vi "visualization_sub_analog.vi"(10 "Latest?":bool, 11 "Instance":i32) -> (2 "ADC_Array":dbl[](array[numeric]), 3 "Analog Data Cluster":T1, 5 "dataToRead?":bool)   [LabVIEW 2022 SP3]
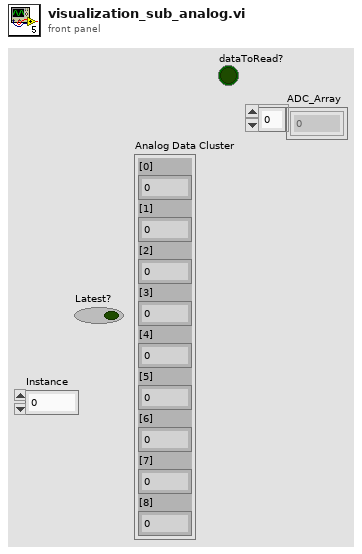
[diagram p1: front panel]
types:
  T1 = cluster{"[0]":dbl, "[1]":dbl, "[2]":dbl, "[3]":dbl, "[4]":dbl, "[5]":dbl, "[6]":dbl, "[7]":dbl, "[8]":dbl}
  T2 = cluster{"ADC_Array[0]":dbl, "ADC_Array[1]":dbl, "ADC_Array[2]":dbl, "ADC_Array[3]":dbl, "ADC_Array[4]":dbl, "ADC_Array[5]":dbl, "ADC_Array[6]":dbl, "ADC_Array[7]":dbl, "ADC_Array[8]":dbl}
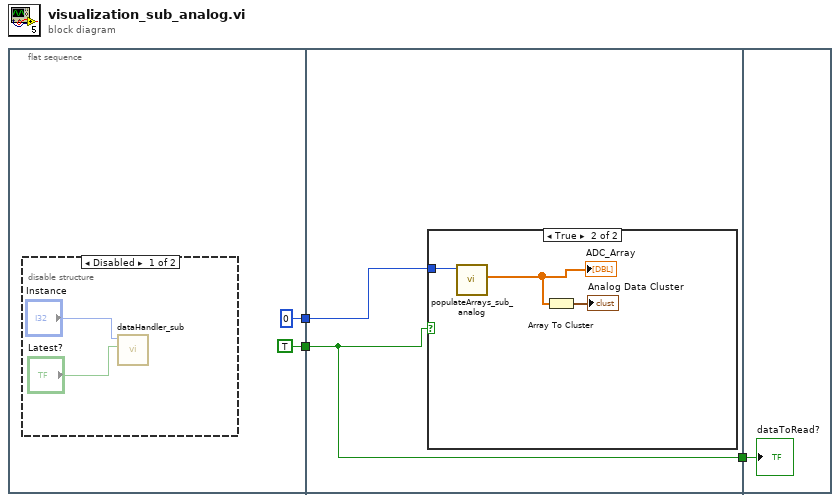
[diagram p0: block diagram]
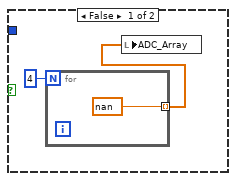
[diagram p3: hidden frame]
diagram:
  n1 = flat-sequence {
    tunnel: [0 ("Instance")] -> w3
    tunnel: [TRUE ("dataToRead?")] -> w2
    tunnel: w3 -> [w9]
    tunnel: w2 -> [w8]
    tunnel: [w8] -> w1
    tunnel: w1 -> [w16]
    frame #0 {
      n2 = disable-structure shown="Disabled" {
        frame Disabled {
          n3 = call "dataHandler_sub.vi"("Instance"="Instance", "Latest?"="Latest?") -> ()  [unwired: 7 in, 2 out]
        }
        frame Enabled {
        }
      }
    }
    frame #1 {
      n4 = case shown="True" w8 {
        tunnel: w9 -> [_ w15]
        frame False {
          n5 = for {
            N: 4 -> [_]
            tunnel: [nan] -> w10 mode=indexing
          }
          n6 = local write "ADC_Array"(w10) -> ()
        }
        frame True {
          n7 = call "populateArrays_sub_analog.vi"("Instance"=w15) -> ("ADC_Array"=w13:dbl[])  [unwired: 10 in]
          "ADC_Array" <- w13
          n8 = Array To Cluster(array=w13) -> (cluster=→"Analog Data Cluster":T2)
        }
      }
    }
    frame #2 {
      "dataToRead?" <- w16
    }
  }
